vi "Ejercicio 1.2.vi"() -> ()   [LabVIEW 2020]
panel:
  in  "Cantidad":dbl(slide) scale=0.0..10.0
  out "Cantidad":dbl(knob) scale=0.0..10.0
  out "Encender":bool
  in  "Encender":bool
  out "Nombre":string
  in  "Nombre":string
  out "Edad":dbl(slide) scale=0.0..30.0
  in  "Edad":dbl
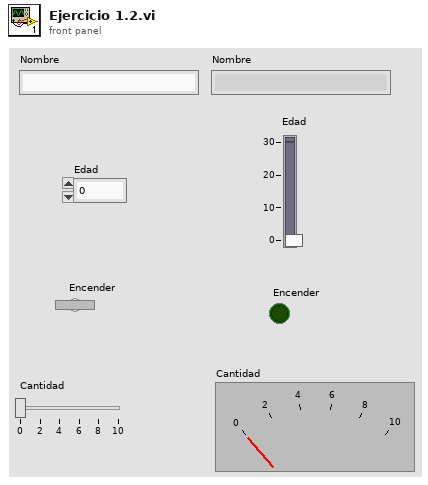
[diagram p1: front panel]
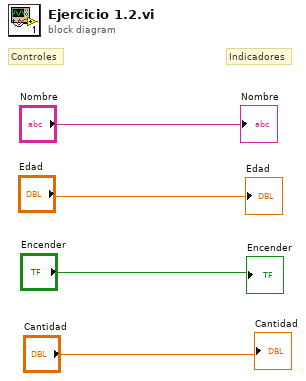
[diagram p0: block diagram]
diagram:
  # "Indicadores"
  # "Controles"
  "Edad" <- "Edad"
  "Nombre" <- "Nombre"
  "Encender" <- "Encender"
  "Cantidad" <- "Cantidad"
